vi "AnalogFilter.vi"(1 "Window Size":i32, 2 "Analog Input":dbl) -> (0 "Analog Output":dbl)   [LabVIEW 2020]
doc: "Takes inpute from an analog sensor and averageds inputs over the window (Window Size)"
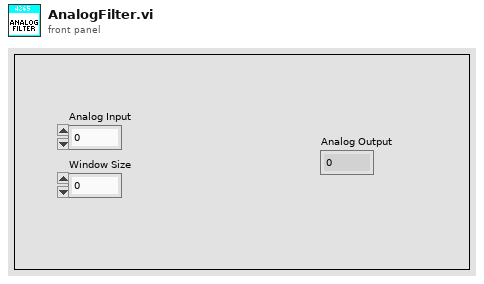
[diagram p1: front panel]
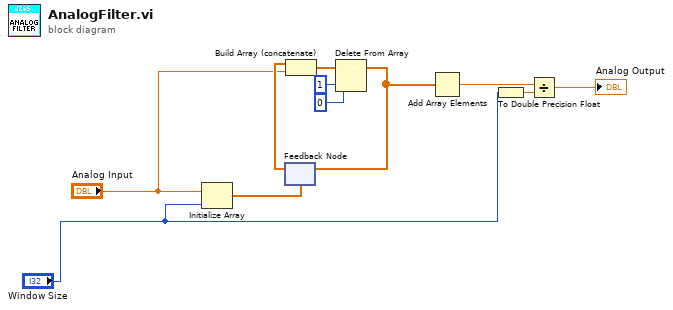
[diagram p0: block diagram]
diagram:
  n1 = Initialize Array("Analog Input", "Window Size") -> (w11:dbl[])
  n2 = feedback #1(w11) -> (w10:dbl[])
  n3 = Build Array (concatenate)(w10, "Analog Input") -> (w8:dbl[])
  n4 = Delete From Array(array=w8, length=1, index=0) -> (array with subset deleted=w5:dbl[])  [unwired: 1 out]
  n5 = feedback-in #1(w5) -> ()
  n6 = Add Array Elements(numeric array=w5) -> (sum=w4:dbl)
  n7 = To Double Precision Float(number="Window Size") -> (double precision float=w2:dbl)
  n8 = Divide(x=w4, y=w2) -> (x/y=→"Analog Output":dbl)
